vi "Verify if the output is on.vi"(8 "error in (no error)":errorcluster, 10 "Output":string, 11 "Sync Box in":refnum<class "Sync Box.lvclass">) -> (0 "error out":errorcluster, 2 "Is output ON ?":bool, 3 "Sync Box out":refnum<class "Sync Box.lvclass">)   [LabVIEW 2018, in "Sync Box.lvclass"]
uses:
  Sync Box.lvclass
  Sync Box.lvclass/Sync Box.ctl
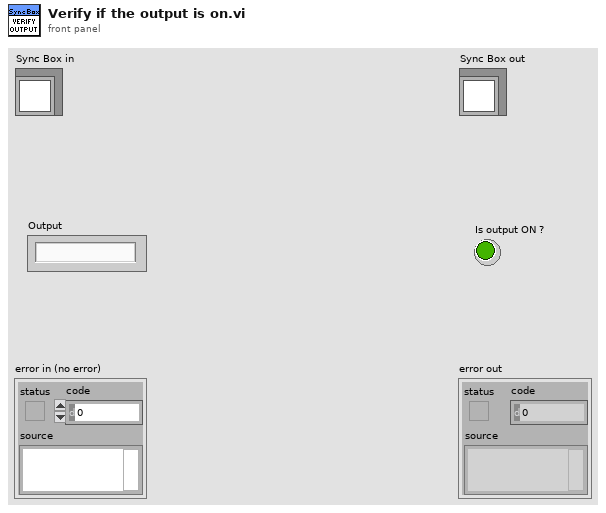
[diagram p1: front panel]
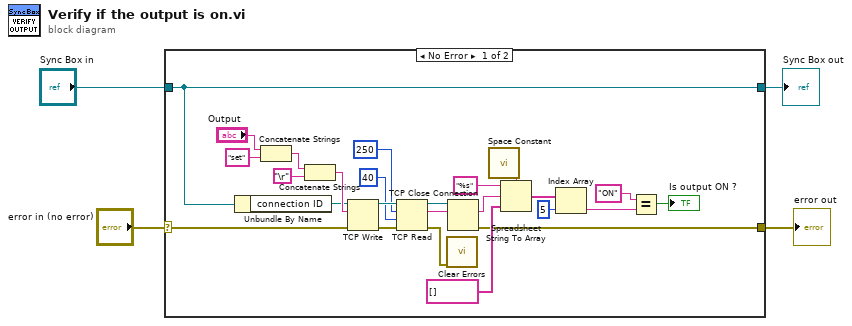
[diagram p0: block diagram]
diagram:
  n1 = case shown="No Error" "error in (no error)" {
    selector: "error in (no error)" -> [w9 w30]
    tunnel: [w8 w30] -> w3
    tunnel: [w11 w29] -> w1
    tunnel: "Sync Box in" -> [w11 w29]
    frame No Error {
      n2 = Unbundle By Name(w11) -> ("connection ID"=w10:refnum<k5>)
      n3 = Concatenate Strings("Output", "set") -> (w7:string)
      n4 = Concatenate Strings(w7, "\r") -> (w28:string)
      n5 = TCP Write(connection ID=w10, data in=w28, error in (no error)=w9) -> (connection ID out=w25:refnum<k5>, error out=w26:errorcluster)  [unwired: 1 in, 1 out]
      n6 = TCP Read(connection ID=w25, bytes to read=250, error in (no error)=w26, 9:40 ("timeout ms (25000)")) -> (connection ID out=w24:refnum<k5>, data out=w20:string, error out=w21:errorcluster)  [unwired: 1 in]
      n7 = call <vilib>:"Clear Errors.vi"("error in (no error)"=w21) -> ()  [unwired: 5 in, 2 out]
      n8 = TCP Close Connection(connection ID=w24) -> (error out=w8:errorcluster)  [unwired: 2 in, 1 out]
      n9 = call <vilib>:"Space Constant.vi"() -> ("String"=w17:string)
      n10 = Spreadsheet String To Array(delimiter (Tab)=w17, format string="%s", spreadsheet string=w20, array type (2D Dbl)=string[] []) -> (array=w15:string[])
      n11 = Index Array(array=w15, index=5) -> (element=w14:string)
      n12 = Equal?(x="ON", y=w14) -> (x = y?=→"Is output ON ?":bool)
    }
    frame Error {
    }
  }
  "error out" <- w3
  "Sync Box out" <- w1
